vi "xwpfDocument Tests Append To File.vi"() -> ()   [LabVIEW 2017]
uses:
  src/LabVIEW NPOI/xwpfDocument/xwpfDocument.lvclass/xwpfDocument.ctl
  src/LabVIEW NPOI/xwpfDocument/Get Elements.Text.vi
  src/LabVIEW NPOI/xwpfDocument.Element/xwpfDocument.Element.lvclass
  src/LabVIEW NPOI/xwpfDocument/xwpfDocument.lvclass
panel:
  out "Elements":string[](array[string])
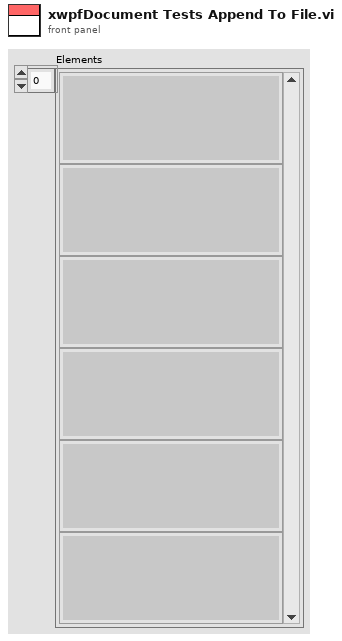
[diagram p1: front panel]
types:
  T1 = enum16{"Title", "Heading 1", "Heading 2", "Heading 3", "Normal", "Figure", "Page Break"}[]
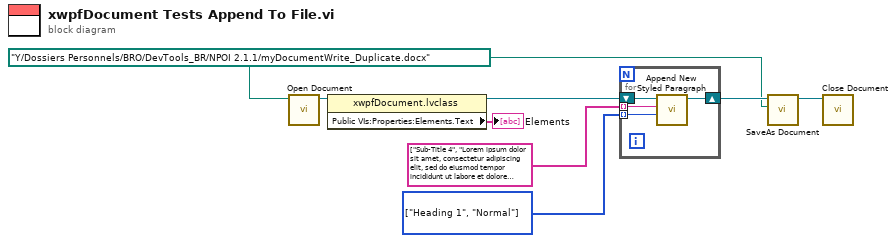
[diagram p0: block diagram]
diagram:
  w4 = T1 [enum."Heading 1", enum."Normal"] items=["Title", "Heading 1", "Heading 2", "Heading 3", "Normal", "Figure", "Page Break"]
  w1 = path "Y:/Dossiers Personnels/BRO/DevTools_BR/NPOI 2.1.1/myDocumentWrite_Duplicate.docx" ("Document Path")
  n1 = call "Open Document.vi"("Document Path"=w1) -> ("xwpfDocument out"=w8:refnum<class "xwpfDocument.lvclass">)  [unwired: 9 in, 1 out]
  n2 = property class="xwpfDocument.lvclass"(reference=w8) -> (reference out=w6:refnum<class "xwpfDocument.lvclass">, "Public VIs:Properties:Elements.Text"=→"Elements":string[])  [unwired: 1 in, 1 out]
  n3 = for {
    shift-right: [w11] -> w3
    shift-left: w6 -> [w12]
    tunnel: string[] ["Sub-Title 4", "Lorem ipsum dolor sit amet, consectetur adipiscing elit, sed do eiusmod tempor incididunt ut labore et dolore magna aliqua. Aliquam purus sit amet luctus venenatis lectus magna fringilla urna. Egestas sed sed risus pretium quam vulputate dignissim suspendisse. Donec enim diam vulputate ut pharetra. Quis commodo odio aenean sed. Nisi vitae suscipit tellus mauris a. Aenean sed adipiscing diam donec adipiscing tristique risus nec. Egestas sed sed risus pretium quam vulputate dignissim. Massa placerat duis ultricies lacus. Nec feugiat nisl pretium fusce id velit ut tortor pretium. Tincidunt tortor aliquam nulla facilisi cras fermentum odio eu feugiat. Feugiat sed lectus vestibulum mattis ullamcorper velit sed ullamcorper. Pulvinar mattis nunc sed blandit libero volutpat. Pulvinar elementum integer enim neque volutpat ac tincidunt vitae."] -> [w10] mode=indexing
    tunnel: w4 -> [w9] mode=indexing
    n4 = call "Append New Styled Paragraph.vi"("Type"=w9, "Paragraph.Text"=w10, "xwpfDocument in"=w12) -> ("xwpfDocument out"=w11:refnum<class "xwpfDocument.lvclass">)  [unwired: 7 in, 1 out]
  }
  n5 = call "SaveAs Document.vi"("Document Path"=w1, "xwpfDocument in"=w3) -> ("xwpfDocument out"=w2:refnum<class "xwpfDocument.lvclass">)  [unwired: 8 in, 1 out]
  n6 = call "Close Document.vi"("xwpfDocument in"=w2) -> ()  [unwired: 9 in, 2 out]
